vi "EFuse settings to Register to Write Array.vi"(8 "error in (no error)":errorcluster, 11 "Toggle 6 in":refnum<class "Toggle 7.1.lvclass">) -> (0 "error out":errorcluster, 1 "Efuse Register Array":T2[](array[typedef]), 2 "Efuse Array":T1[](array[typedef]), 3 "Toggle 6 out":refnum<class "Toggle 7.1.lvclass">)   [LabVIEW 2020, in "Toggle 7.1.lvclass"]
uses:
  Toggle 7.1.lvclass
  Controls/Register to Write.ctl
  Controls/EFuse modes enum.ctl
  PIC-device/PIC-Device.lvclass
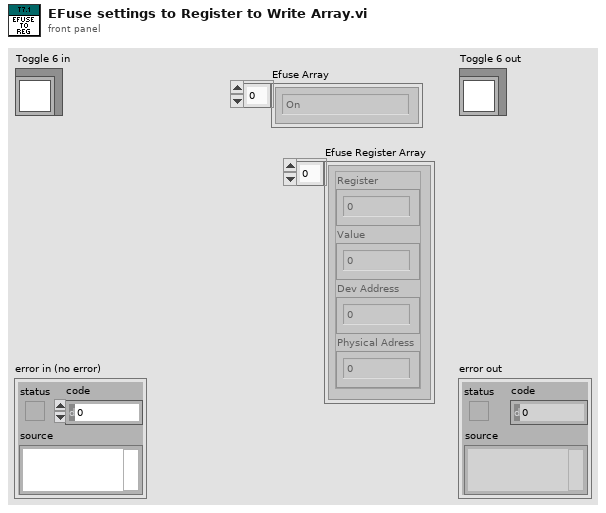
[diagram p1: front panel]
types:
  T1 = typedef "Toggle 7.1.lvclass/EFuse modes enum.ctl" = enum16{"On", "Off", "Both On and Off"}
  T2 = typedef "PIC-Device.lvclass/Register to Write.ctl" = cluster{"Register":u32, "Value":u32, "Dev Address":u32, "Physical Adress":u32}
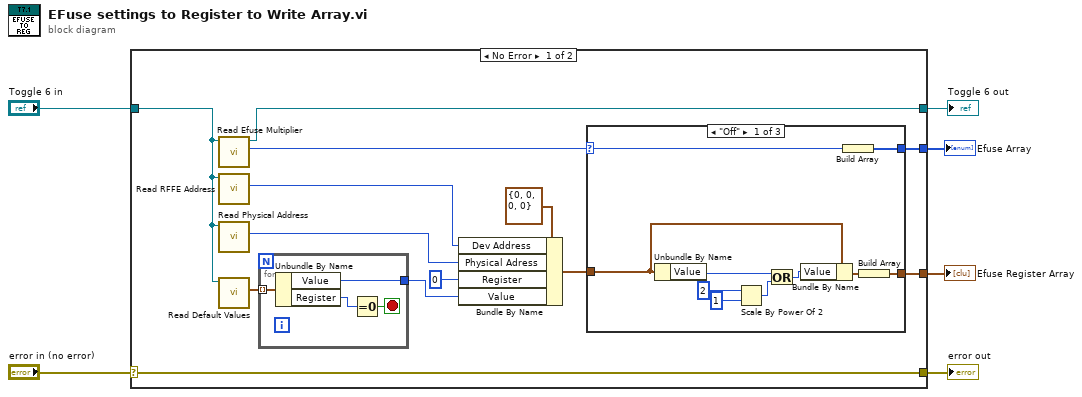
[diagram p0: block diagram]
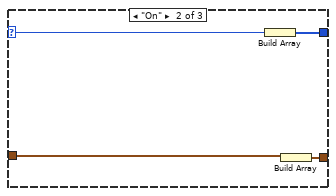
[diagram p2: hidden frame]
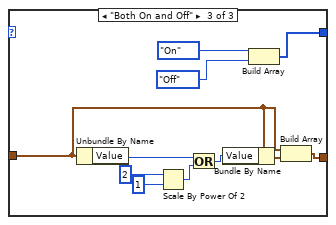
[diagram p3: hidden frame]
diagram:
  n1 = case shown="No Error" "error in (no error)" {
    selector: "error in (no error)" -> [w19 w50]
    tunnel: [w19 w50] -> w5
    tunnel: [w17 w49] -> w3
    tunnel: "Toggle 6 in" -> [w12 w49]
    tunnel: [w8 _] -> w2
    tunnel: [w7 _] -> w1
    frame No Error {
      n2 = call-dynamic "Read Efuse Multiplier.vi"("Toggle 6 in"=w12) -> ("Efuse Multiplier"=w18:T1, "Toggle 6 out"=w17:refnum<class "Toggle 7.1.lvclass">)  [unwired: 9 in]
      n3 = call-dynamic "Read RFFE Address.vi"("Toggle 6 in"=w12) -> ("RFFE Adress"=w15:u32)  [unwired: 8 in, 2 out]
      n4 = call-dynamic "Read Physical Address.vi"("Toggle 6 in"=w12) -> ("Physical Adress"=w14:u32)  [unwired: 9 in, 1 out]
      n5 = call-dynamic "Read Default Values.vi"("Toggle 7.1 in"=w12) -> ("Default Values"=w11:T2[])  [unwired: 9 in, 1 out]
      n6 = for {
        tunnel: w11 -> [w23] mode=indexing
        tunnel: [w20] -> w10
        stop <- w21 stop-if-true
        n7 = Unbundle By Name(w23) -> ("Value"=w20:u32, "Register"=w22:u32)
        n8 = Equal To 0?(x=w22) -> (x = 0?=w21:bool)
      }
      n9 = Bundle By Name(cluster=T2 {"Register"=0, "Value"=0, "Dev Address"=0, "Physical Adress"=0} ("Register to Write"), "Dev Address"=w15, "Physical Adress"=w14, "Register"=u32 0, "Value"=w10) -> (w9:T2)
      n10 = case shown="\"Off\"" w18 {
        selector: w18 -> [w25 w35 _]
        tunnel: w9 -> [w33 w37 w41]
        tunnel: [w26 w36 w42] -> w8
        tunnel: [w24 w34 w40] -> w7
        frame "Off" {
          n11 = Unbundle By Name(w33) -> ("Value"=w32:u32)
          n12 = Scale By Power Of 2(n=i16 2, x=u32 1) -> (x*2^n=w31:u32)
          n13 = Or(x=w32, y=w31) -> (x .or. y?=w28:u32)
          n14 = Bundle By Name(cluster=w33, "Value"=w28) -> (w27:T2)
          n15 = Build Array(w25) -> (w24:T1[])
          n16 = Build Array(w27) -> (w26:T2[])
        }
        frame "On" {
          n17 = Build Array(w35) -> (w34:T1[])
          n18 = Build Array(w37) -> (w36:T2[])
        }
        frame "Both On and Off" {
          n19 = Unbundle By Name(w41) -> ("Value"=w48:u32)
          n20 = Scale By Power Of 2(n=i16 2, x=u32 1) -> (x*2^n=w47:u32)
          n21 = Or(x=w48, y=w47) -> (x .or. y?=w44:u32)
          n22 = Bundle By Name(cluster=w41, "Value"=w44) -> (w43:T2)
          n23 = Build Array(EFuse_modes_enum."On" ("Efuse Multiplier"), EFuse_modes_enum."Off" ("Efuse Multiplier")) -> (w40:T1[])
          n24 = Build Array(w41, w43) -> (w42:T2[])
        }
      }
    }
    frame Error {
    }
  }
  "error out" <- w5
  "Toggle 6 out" <- w3
  "Efuse Register Array" <- w2
  "Efuse Array" <- w1
